vi "8-bit video export-Progress string.vi"(7 "Currnet frame number in selected chunk (1based)":i32, 9 "Exporting":bool, 11 "Number of frames in selected chunk":i32) -> (3 "Progress string":string)   [LabVIEW 2017]
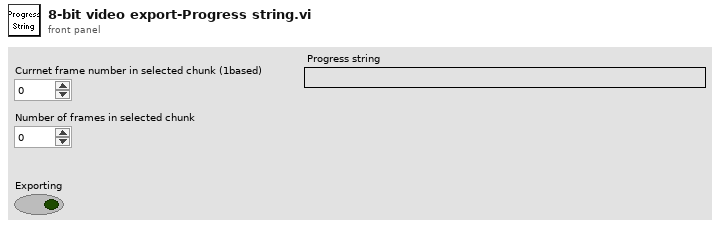
[diagram p1: front panel]
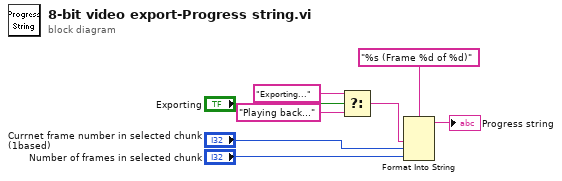
[diagram p0: block diagram]
diagram:
  n1 = Select(t="Exporting..." ("initial string"), s="Exporting", f="Playing back...") -> (s? t:f=w7:string)
  n2 = Format Into String(format string="%s (Frame %d of %d)", w7, "Currnet frame number in selected chunk (1based)", "Number of frames in selected chunk") -> (resulting string=→"Progress string":string)  [unwired: 2 in, 1 out]
